vi "ReadAccels.vi"(8 "error in":errorcluster, 11 "Data":T2={"FPGARef"=refnum, "Data Rate(Hz)"=0.0, "Sensitivities(mv/(m/s2))"=[0.0, 0.0, 0.0, 0.0], "Cutoff Frequncies"=[], "Waterfall Select"=0} {"Cutoff Frequncies"."HP Passband" min=1.0 step=1.0 format="%#.4f"; "Cutoff Frequncies"."LP Stopband" min=1.0 step=1.0 format="%#.4f"; "Cutoff Frequncies"."HP Stopband" min=1.0 step=1.0 format="%#.4f"; "Cutoff Frequncies"."LP Passband" min=1.0 step=1.0 format="%#.4f"}) -> (0 "error out":errorcluster)   [LabVIEW 2018, in "Vibration.lvlib"]
uses:
  Vibration.lvlib
  Private Controls/Host Comms Data.ctl
  FPGA/FPGA VI Reference.ctl
  Modules/Testing UI 3/Private Controls/Cutoff Frequency.ctl
  <vilib>/addons/Sound and Vibration/svt_Calibration/SVL Scale Voltage to EU.vi
  <vilib>/addons/Sound and Vibration/svt_Calibration/SVL Scale Voltage to EU (1 Ch).vi
  <vilib>/addons/_NISVFA/_Shared subVIs/Common/svc_Set SV Channel Info.vi
  <vilib>/addons/_NISVFA/_Shared subVIs/Common/svc_Set SV Channel Info (variant).vi
  <vilib>/addons/_NISVFA/_Shared subVIs/Common/SVL Set dB Reference (variant).vi
  <vilib>/Utility/error.llb/Error Cluster From Error Code.vi
  <vilib>/rvi/errors/niLvFpgaAdjustHostInterfaceError.vi
  <vilib>/addons/_NISVFA/_Shared subVIs/Common/svc_Engineering Units to Unit Label.vi
  <vilib>/addons/_NISVFA/_Shared subVIs/Common/svc_Compute Scale Factor to Convert V to EU.vi
  <vilib>/addons/_NISVFA/_Shared subVIs/Common/svc_Compute Scale Factor to Convert C to EU.vi
  <vilib>/addons/_NISVFA/_Shared subVIs/Common/svc_Set dB ref if Pascal.vi
  <vilib>/addons/_NISVFA/_Shared subVIs/Common/svc_Caller VI Returned in Error Source.vi
  <vilib>/addons/Sound and Vibration/Order Analysis/Referece Data Processing/OAT FIR Preprocess Filter.vi
  <vilib>/addons/Sound and Vibration/Order Analysis/Referece Data Processing/OAT FIR Preprocess Filter (1 Channel).vi
  <vilib>/addons/Sound and Vibration/svt_Level/SVL RMS Level.vi
  <vilib>/addons/Sound and Vibration/svt_Level/SVL RMS Level (1 Ch).vi
  <vilib>/addons/Sound and Vibration/svt_Integration/SVL Integration.vi
  <vilib>/addons/Sound and Vibration/svt_Integration/SVL Integration (1 Ch).vi
  <vilib>/addons/Sound and Vibration/svt_Level/SVL Peak Level.vi
  <vilib>/addons/Sound and Vibration/svt_Level/SVL Peak Level (1 Ch).vi
  <vilib>/rvi/interface/nirviMethod/nirviMethod.xnode
  <vilib>/FPGAPlugInAG/Dynamic/niLvFpga_ReadFifo_Dynamic.vi
  <vilib>/rvi/errors/niLvFpgaMergeErrorWithErrorCode.vi
  RT-UDP Writer/UDP Writer.lvlib
  Modules/Testing UI 3/Testing UI 3.lvlib
panel:
  out "Elements Remaining":u32
  out "output cluster":T1
  # "Highpass Cutoff Frequency"
  # "Lowpass Cutoff Frequency"
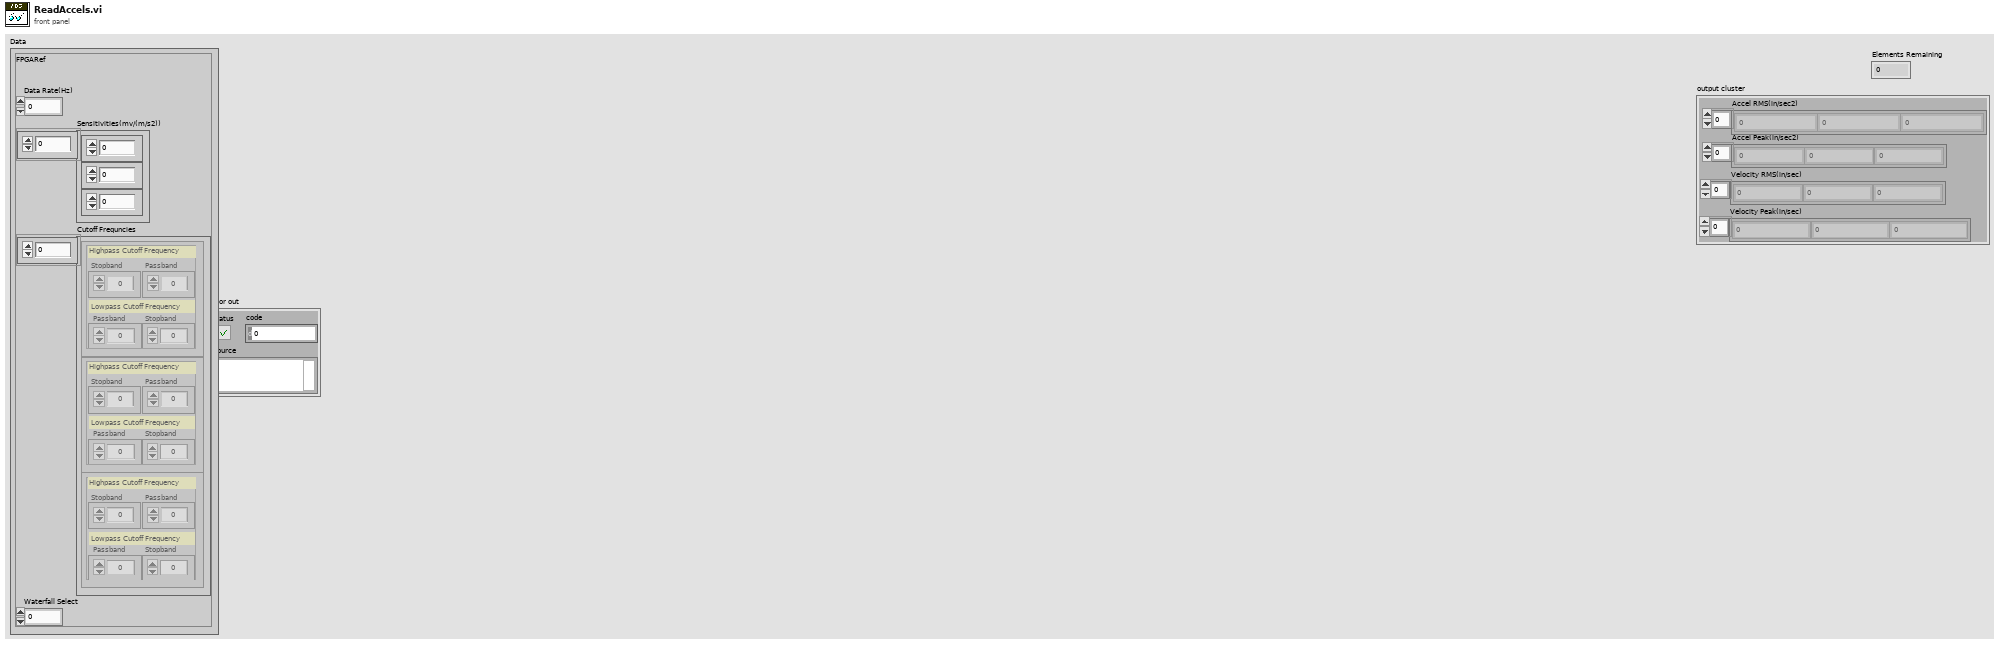
[diagram p1: front panel]
types:
  T1 = cluster{"Accel RMS(in/sec2)":dbl[], "Accel Peak(in/sec2)":dbl[], "Velocity RMS(in/sec)":dbl[], "Velocity Peak(in/sec)":dbl[]}
  T2 = typedef "Vibration.lvlib/Host Comms Data.ctl" = cluster{"FPGARef":T3, "Data Rate(Hz)":dbl, "Sensitivities(mv/(m/s2))":dbl[], "Cutoff Frequncies":T4[], "Waterfall Select":u8}
  T3 = typedef "FPGA VI Reference.ctl" = refnum<k20>
  T4 = typedef "Testing UI 3.lvlib/Cutoff Frequency.ctl" = cluster{"LP Passband":dbl, "HP Stopband":dbl, "LP Stopband":dbl, "HP Passband":dbl}
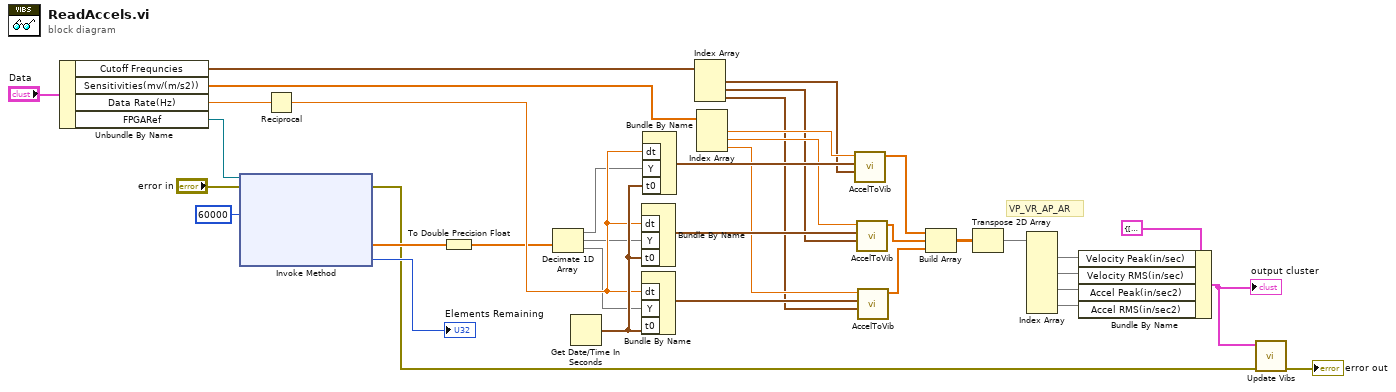
[diagram p0: block diagram]
diagram:
  # "VP_VR_AP_AR"
  n1 = Unbundle By Name("Data") -> ("Cutoff Frequncies"=w34:T4[], "Sensitivities(mv/(m/s2))"=w33:dbl[], "Data Rate(Hz)"=w31:dbl, "FPGARef"=w35:T3)
  n2 = xnode "Invoke Method"("FPGA VI Reference In"=w35, "error in"="error in", "Number of Elements"=u32 60000) -> ("error out"=w2:errorcluster, "Data"=w22:sgl[], "Elements Remaining"=→"Elements Remaining":u32)  [unwired: 1 in, 1 out]
  n3 = Reciprocal(x=w31) -> (1/x=w30:dbl)
  n4 = To Double Precision Float(number=w22) -> (double precision float=w11:dbl[])
  n5 = Decimate 1D Array(w11) -> (w27:dbl[], w26:dbl[], w25:dbl[])
  n6 = Get Date/Time In Seconds() -> (seconds since 1Jan1904=w32:timestamp)
  n7 = Bundle By Name("dt"=w30, "Y"=w26, "t0"=w32) -> (w18:waveform(dbl))  [unwired: 1 out]
  n8 = Bundle By Name("dt"=w30, "Y"=w25, "t0"=w32) -> (w14:waveform(dbl))  [unwired: 1 out]
  n9 = Bundle By Name("dt"=w30, "Y"=w27, "t0"=w32) -> (w21:waveform(dbl))  [unwired: 1 out]
  n10 = Index Array(array=w34) -> (element #1=w19:T4, element #2=w16:T4, element #3=w13:T4)  [unwired: 3 in]
  n11 = Index Array(array=w33) -> (element #1=w20:dbl, element #2=w17:dbl, element #3=w15:dbl)  [unwired: 3 in]
  n12 = call "AccelToVib.vi"("Filters"=w19, "Waveform"=w21, "mV/(m/s2)"=w20) -> ("VP_VR_AP_AR"=w12:dbl[])  [unwired: 7 in, 1 out]
  n13 = call "AccelToVib.vi"("Filters"=w16, "Waveform"=w18, "mV/(m/s2)"=w17) -> ("VP_VR_AP_AR"=w10:dbl[])  [unwired: 7 in, 1 out]
  n14 = call "AccelToVib.vi"("Filters"=w13, "Waveform"=w14, "mV/(m/s2)"=w15) -> ("VP_VR_AP_AR"=w9:dbl[])  [unwired: 7 in, 1 out]
  n15 = Build Array(w12, w10, w9) -> (w8:dbl[][])
  n16 = Transpose 2D Array(2D array=w8) -> (transposed array=w7:dbl[][])
  n17 = Index Array(array=w7) -> (element #1=w6:dbl[], element #2=w5:dbl[], element #3=w4:dbl[], element #4=w3:dbl[])  [unwired: 8 in]
  n18 = Bundle By Name(cluster=T1 {"Accel RMS(in/sec2)"=[], "Accel Peak(in/sec2)"=[], "Velocity RMS(in/sec)"=[], "Velocity Peak(in/sec)"=[]} ("All Data Cluster.Accel Data"), "Velocity Peak(in/sec)"=w6, "Velocity RMS(in/sec)"=w5, "Accel Peak(in/sec2)"=w4, "Accel RMS(in/sec2)"=w3) -> (w29:T1)
  "output cluster" <- w29
  n19 = call "Update Vibs.vi"("error in"=w2, "Accel"=w29) -> ("error out"=→"error out":errorcluster)  [unwired: 9 in]
